vi "Verif Clock 2.vi"(8 "error in (no error)":errorcluster, 10 "period (ms)":u32=500, 11 "State Machine in":refnum<class "State Machine.lvclass">) -> (0 "error out":errorcluster, 2 "time elapsed":u32, 3 "State Machine out":refnum<class "State Machine.lvclass">)   [LabVIEW 2018, in "State Machine.lvclass"]
uses:
  State Machine.lvclass
  State Machine.lvclass/State Machine.ctl
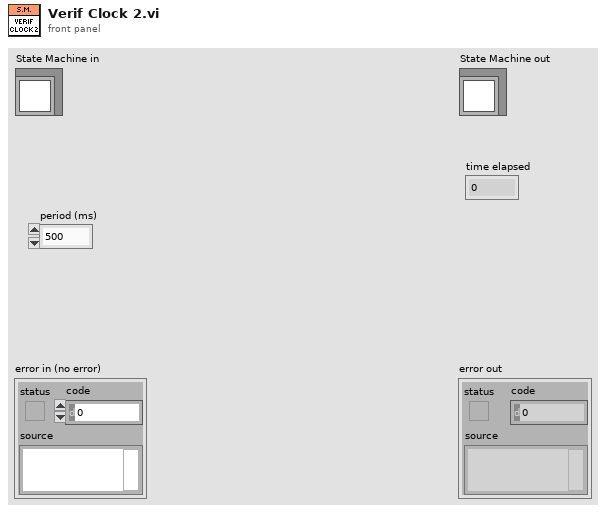
[diagram p1: front panel]
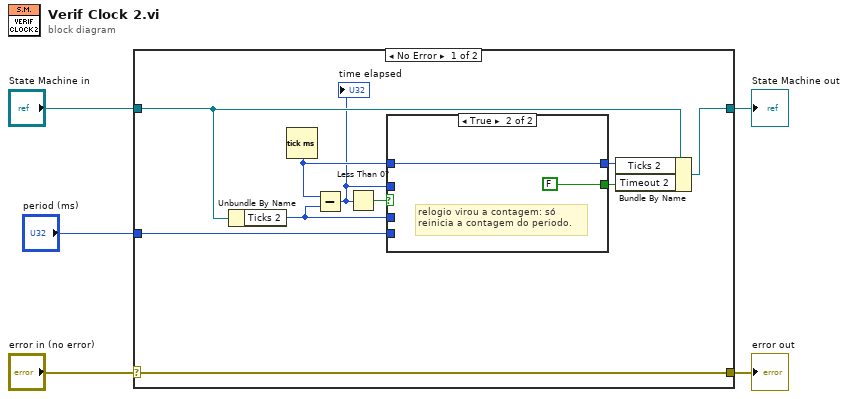
[diagram p0: block diagram]
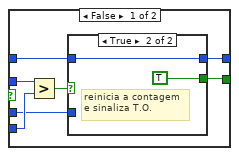
[diagram p2: hidden frame]
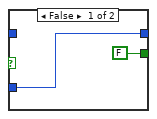
[diagram p3: hidden frame]
diagram:
  n1 = case shown="No Error" "error in (no error)" {
    selector: "error in (no error)" -> [w15 w30]
    tunnel: [w15 w30] -> w4
    tunnel: [w13 w29] -> w2
    tunnel: "State Machine in" -> [w14 w29]
    tunnel: "period (ms)" -> [w9 _]
    frame No Error {
      n2 = Unbundle By Name(w14) -> ("Ticks 2"=w7:u32)
      n3 = Tick Count (ms)() -> (millisecond timer value=w11:u32)
      n4 = Subtract(x=w11, y=w7) -> (x-y=w8:u32)
      "time elapsed" <- w8
      n5 = Less Than 0?(x=w8) -> (x < 0?=w12:bool)
      n6 = case shown="True" w12 {
        tunnel: w11 -> [w19 w28]
        tunnel: [w18 w28] -> w10
        tunnel: [w17 FALSE] -> w6
        tunnel: w9 -> [w22 _]
        tunnel: w8 -> [w21 _]
        tunnel: w7 -> [w16 _]
        frame False {
          n7 = Greater?(x=w21, y=w22) -> (0:w20:bool)
          n8 = case shown="True" w20 {
            tunnel: [w24 w26] -> w18
            tunnel: w19 -> [_ w26]
            tunnel: [FALSE TRUE] -> w17
            tunnel: w16 -> [w24 _]
            frame False {
            }
            frame True {
              # "reinicia a contagem\ne sinaliza T.O."
            }
          }
        }
        frame True {
          # "relogio virou a contagem: só\nreinicia a contagem do periodo."
        }
      }
      n9 = Bundle By Name(cluster=w14, "Ticks 2"=w10, "Timeout 2"=w6) -> (w13:refnum<class "State Machine.lvclass">)
    }
    frame Error {
    }
  }
  "error out" <- w4
  "State Machine out" <- w2
